vi "Crash.vi"(8 "error in (no error)":errorcluster, 11 "Mouse in":refnum<class "Mouse.lvclass">) -> (0 "error out":errorcluster, 3 "Mouse out":refnum<class "Mouse.lvclass">)   [LabVIEW 2020, in "Maze.lvlib" / "Mouse.lvclass"]
doc: "This VI is called to let your mouse know that it has run head-first into a wall. This typically hurts because you are, in fact, a racing mouse and this will end your current run. You shouldn't ever give a <b>Forward</b> action whenever your Forward distance reading value is zero."
uses:
  Mouse.lvclass
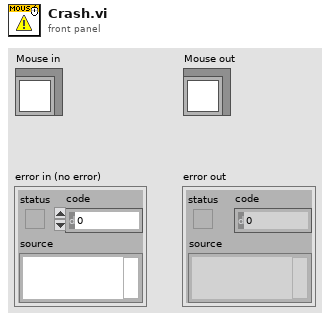
[diagram p1: front panel]
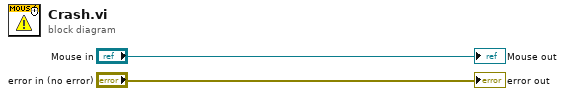
[diagram p0: block diagram]
diagram:
  "error out" <- "error in (no error)"
  "Mouse out" <- "Mouse in"
